vi "WXA100气象仪数据插入.vi"(0 "Tabe Name":string, 1 "data":T1, 3 "错误输入（无错误）":errorcluster) -> (10 "错误输出":errorcluster)   [LabVIEW 2016]
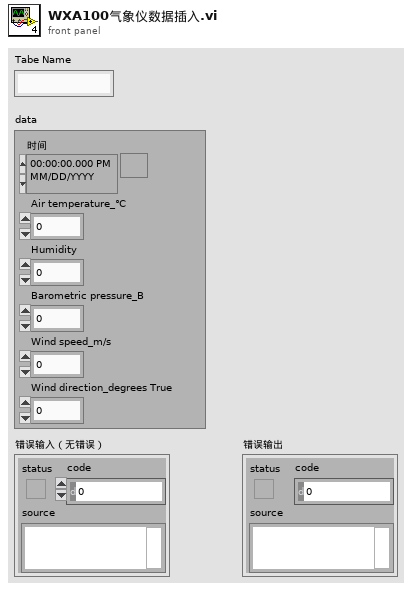
[diagram p1: front panel]
types:
  T1 = typedef "WXA100气象仪字段定义.ctl" = cluster{"时间":timestamp, "Air temperature_℃":sgl, "Humidity":sgl, "Barometric pressure_B":sgl, "Wind speed_m/s":sgl, "Wind direction_degrees True":sgl}
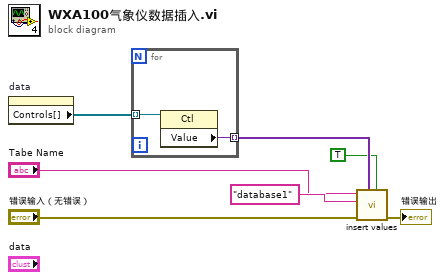
[diagram p0: block diagram]
diagram:
  n1 = property on="data" class="Clust (严格)"() -> ("Controls[]"=w1:refnum<vi>[])  [unwired: 2 in, 2 out]
  n2 = for {
    tunnel: w1 -> [w9] mode=indexing
    tunnel: [w8] -> w7 mode=indexing
    n3 = property class="Ctl"(reference=w9) -> ("Value"=w8:variant)  [unwired: 1 in, 2 out]
  }
  n4 = call "insert values.vi"("是否创建唯一键"=TRUE, "data"=w7, "错误输入（无错误）"="错误输入（无错误）", "database"="database1", "Tabe Name"="Tabe Name") -> ("错误输出"=→"错误输出":errorcluster)  [unwired: 6 in]
